vi "eGateHSP_LoadChannelInfo.vi"(7 "path in":path, 8 "Fehler (Eingang, kein Fehler)":errorcluster, 11 "e.gate Configuration":T1 {"StartTime" format="%#.10f"; "dActTimeToSecondFactor" format="%#.10f"; "StartTimeToDayFactor" format="%#_10f"}) -> (0 "Fehler (Ausgang)":errorcluster, 3 "e.gate Configuration 2":T1 {"StartTime" format="%#.10f"; "dActTimeToSecondFactor" format="%#.10f"; "StartTimeToDayFactor" format="%#_10f"})   [LabVIEW 2016]
uses:
  e.gate Configuration.ctl
  e.gate Channel Data.ctl
  e.gate Data Type.ctl
  e.gate Protocol Type.ctl
  e.gate Module  Data.ctl
  e.gateHSP_DLLhandle.ctl
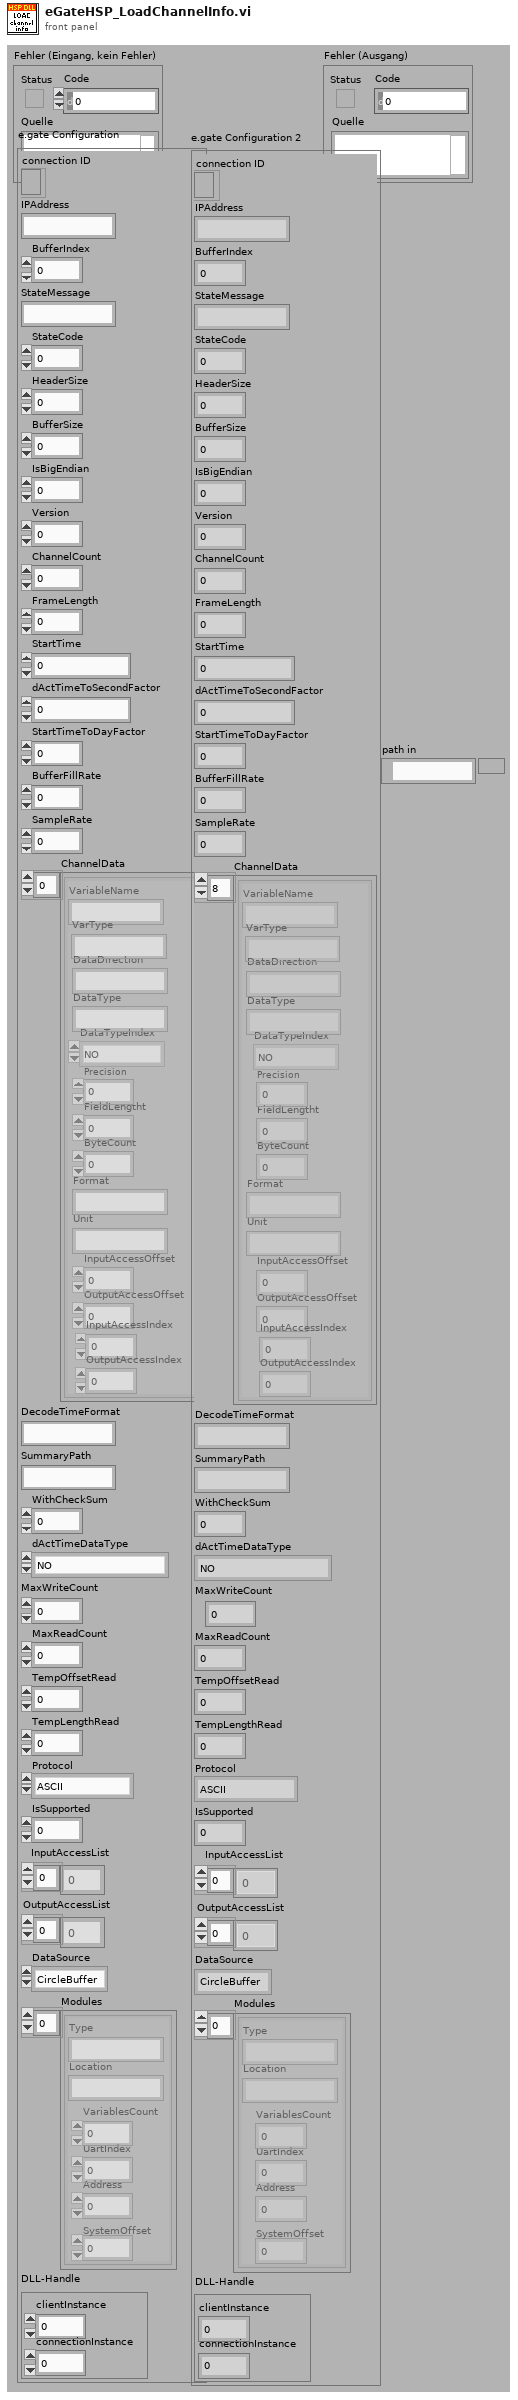
[diagram p1: front panel]
types:
  T1 = typedef "e.gate Configuration.ctl" = cluster{"connection ID":refnum<k5>, "IPAddress":string, "BufferIndex":i32, "StateMessage":string, "StateCode":i8, "HeaderSize":i32, "BufferSize":i32, "IsBigEndian":i32, "Version":i32, "ChannelCount":i32, "FrameLength":i32, "StartTime":dbl, "dActTimeToSecondFactor":dbl, "StartTimeToDayFactor":dbl, "BufferFillRate":dbl, "SampleRate":dbl, "ChannelData":T2[], "DecodeTimeFormat":string, "SummaryPath":string, "WithCheckSum":i32, "dActTimeDataType":T3, "MaxWriteCount":i32, "MaxReadCount":i32, "TempOffsetRead":i32, "TempLengthRead":i32, "Protocol":T4, "IsSupported":i32, "InputAccessList":i32[], "OutputAccessList":i32[], "DataSource":enum16{"CircleBuffer", "test.con Logger", "test.con Archive"}, "Modules":T5[], "DLL-Handle":T6}
  T2 = typedef "e.gate Channel Data.ctl" = cluster{"VariableName":string, "DataDirection":string, "DataType":string, "DataTypeIndex":T3, "Precision":i16, "FieldLengtht":i16, "ByteCount":i32, "Format":string, "Unit":string, "InputAccessOffset":i32, "OutputAccessOffset":i16, "InputAccessIndex":i16, "OutputAccessIndex":i16, "VarType":string}
  T3 = typedef "e.gate Data Type.ctl" = enum16{"NO", "BOOL", "SINT8", "USINT8", "SINT16", "USINT16", "SINT32", "USINT32", "FLOAT", "SET8", "SET16", "SET32", "DOUBLE", "SINT64", "USINT64", "SET64"}
  T4 = typedef "e.gate Protocol Type.ctl" = enum16{"ASCII", "HighspeedPort Online", "HighspeedPort Buffer", "eGateHighspeedPortDLL "}
  T5 = typedef "e.gate Module  Data.ctl" = cluster{"Type":string, "Location":string, "VariablesCount":i16, "UartIndex":i16, "Address":i16, "SystemOffset":i16}
  T6 = typedef "e.gateHSP_DLLhandle.ctl" = cluster{"clientInstance":i32, "connectionInstance":i32}
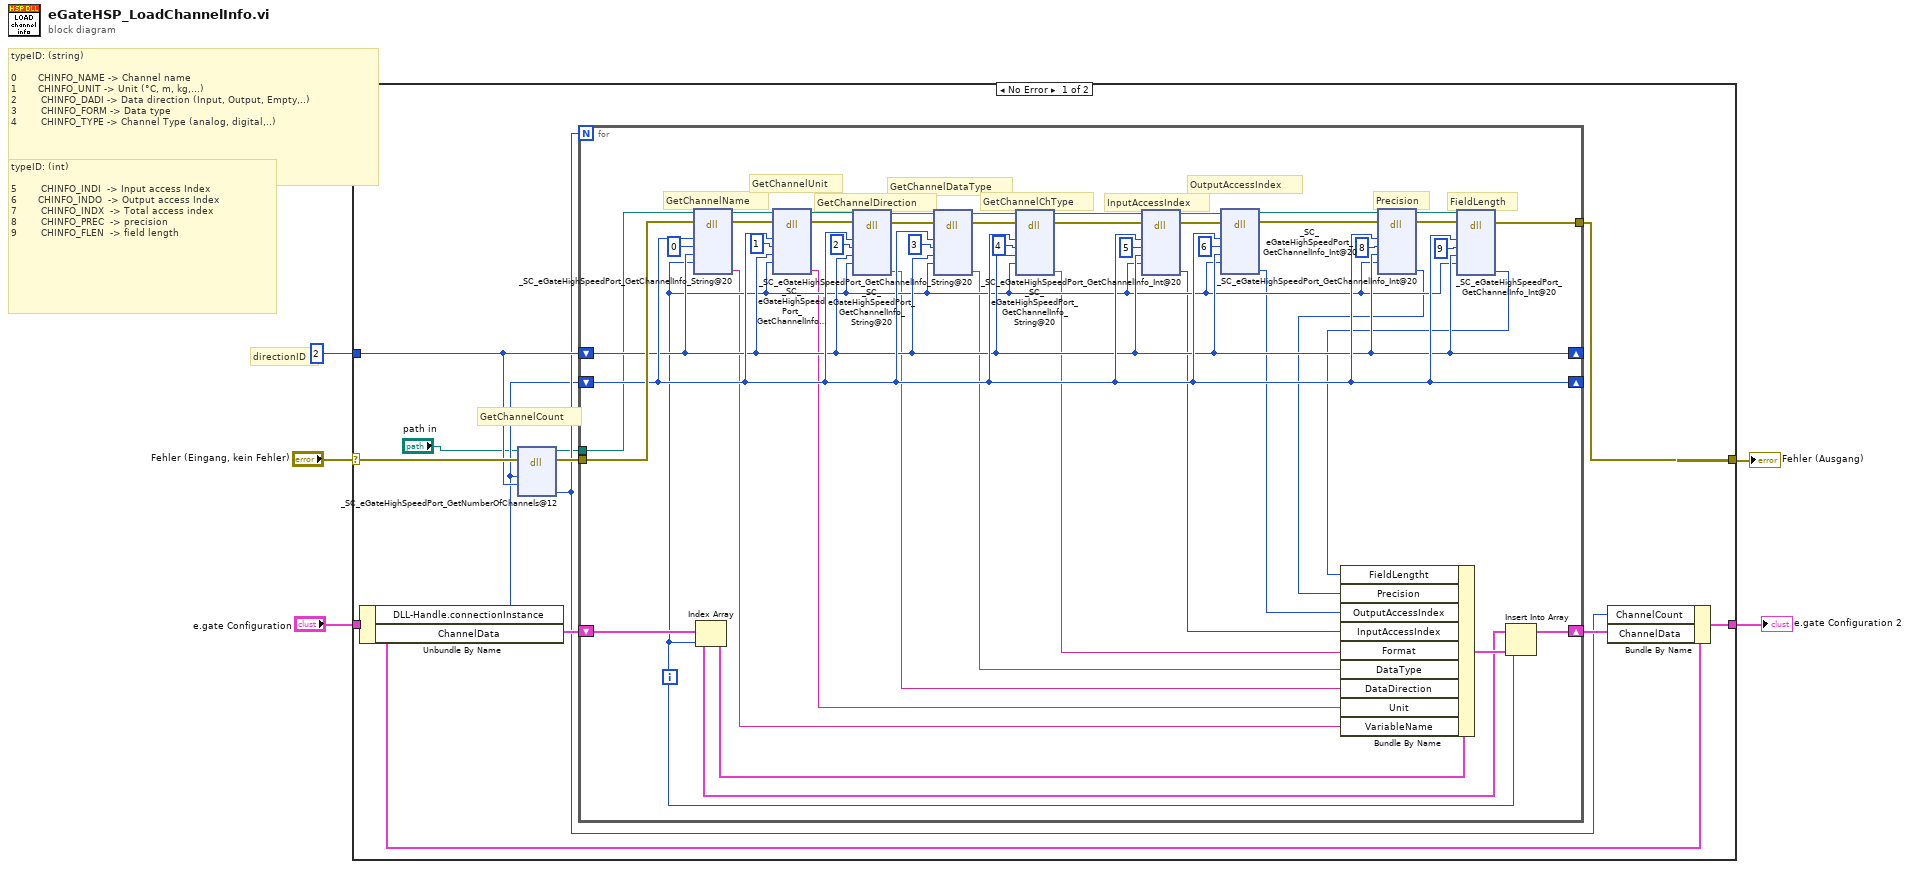
[diagram p0: block diagram]
diagram:
  # "directionID"
  # "typeID: (int)\n\n5\t\t\t\t\t\t\t\tCHINFO_INDI\t\t-> Input access Index\n6\t\t\t\t\t\t\tCHINFO_INDO\t\t-> Output access Index\n7\t\t\t\t\t\t\t\tCHINFO_INDX\t\t-> Total access index\n8\t\t\t\t\t\t\t\tCHINFO_PREC\t\t-> precision\n9\t\t\t\t\t\t\t\tCHINFO_FLEN\t\t-> field length"
  # "typeID: (string)\n\n0\t\t\t\t\t\t\tCHINFO_NAME\t-> Channel name\n1\t\t\t\t\t\t\tCHINFO_UNIT\t-> Unit (°C, m, kg,...)\t\n2\t\t\t\t\t\t\t\tCHINFO_DADI\t-> Data direction (Input, Output, Empty,..)\n3\t\t\t\t\t\t\t\tCHINFO_FORM\t-> Data type\n4\t\t\t\t\t\t\t\tCHINFO_TYPE\t-> Channel Type (analog, digital,..)"
  n1 = case shown="No Error" "Fehler (Eingang, kein Fehler)" {
    selector: "Fehler (Eingang, kein Fehler)" -> [w17 w62]
    tunnel: [w13 w62] -> w4
    tunnel: 2 ("directionID") -> [w14 _]
    tunnel: "e.gate Configuration" -> [w11 _]
    tunnel: [w10 _] -> w2
    frame No Error {
      # "GetChannelCount"
      n2 = Unbundle By Name(w11) -> ("DLL-Handle.connectionInstance"=w8:i32, "ChannelData"=w16:T2[])
      n3 = dll-call lib="eGateHighSpeedPort.dll" fn="_SC_eGateHighSpeedPort_GetNumberOfChannels@12"(path in="path in", error in=w17, "connectionInstance"=w8, "directionID"=w14) -> (path out=w6:path, error out=w15:errorcluster, "ChannelCount"=w9:i32)  [unwired: 5 in]
      n4 = for {
        N: w9 -> [_]
        shift-right: [w59] -> w12
        shift-left: w16 -> [w58]
        tunnel: w15 -> [w51]
        shift-right: [w39] -> _
        shift-left: w8 -> [w39]
        shift-right: [w38] -> _
        shift-left: w14 -> [w38]
        tunnel: [w44] -> w13
        tunnel: w6 -> [w26]
        i -> [w37]
        # "FieldLength"
        # "Precision"
        # "OutputAccessIndex"
        # "InputAccessIndex"
        # "GetChannelChType"
        # "GetChannelDataType"
        # "GetChannelDirection"
        # "GetChannelUnit"
        # "GetChannelName"
        n5 = dll-call lib="eGateHighSpeedPort.dll" fn="_SC_eGateHighSpeedPort_GetChannelInfo_String@20"(path in=w26, error in=w51, "connectionInstance"=w39, "typeID"=0, "directionID"=w38, "channelIndex"=w37) -> (path out=w25:path, error out=w56:errorcluster, "ChannelInfo"=w35:string)  [unwired: 7 in]
        n6 = Index Array(array=w58, index=w37) -> (element=w61:T2)
        n7 = dll-call lib="eGateHighSpeedPort.dll" fn="_SC_eGateHighSpeedPort_GetChannelInfo_String@20"(path in=w25, error in=w56, "connectionInstance"=w39, "typeID"=1, "directionID"=w38, "channelIndex"=w37) -> (path out=w24:path, error out=w50:errorcluster, "ChannelInfo"=w34:string)  [unwired: 7 in]
        n8 = dll-call lib="eGateHighSpeedPort.dll" fn="_SC_eGateHighSpeedPort_GetChannelInfo_String@20"(path in=w24, error in=w50, "connectionInstance"=w39, "typeID"=2, "directionID"=w38, "channelIndex"=w37) -> (path out=w23:path, error out=w49:errorcluster, "ChannelInfo"=w33:string)  [unwired: 7 in]
        n9 = dll-call lib="eGateHighSpeedPort.dll" fn="_SC_eGateHighSpeedPort_GetChannelInfo_String@20"(path in=w23, error in=w49, "connectionInstance"=w39, "typeID"=3, "directionID"=w38, "channelIndex"=w37) -> (path out=w22:path, error out=w48:errorcluster, "ChannelInfo"=w32:string)  [unwired: 7 in]
        n10 = dll-call lib="eGateHighSpeedPort.dll" fn="_SC_eGateHighSpeedPort_GetChannelInfo_String@20"(path in=w22, error in=w48, "connectionInstance"=w39, "typeID"=4, "directionID"=w38, "channelIndex"=w37) -> (path out=w21:path, error out=w47:errorcluster, "ChannelInfo"=w31:string)  [unwired: 7 in]
        n11 = dll-call lib="eGateHighSpeedPort.dll" fn="_SC_eGateHighSpeedPort_GetChannelInfo_Int@20"(path in=w21, error in=w47, "connectionInstance"=w39, "typeID"=5, "directionID"=w38, "channelIndex"=w37) -> (path out=w20:path, error out=w46:errorcluster, "ChannelInfo"=w30:i32)  [unwired: 7 in]
        n12 = dll-call lib="eGateHighSpeedPort.dll" fn="_SC_eGateHighSpeedPort_GetChannelInfo_Int@20"(path in=w20, error in=w46, "connectionInstance"=w39, "typeID"=6, "directionID"=w38, "channelIndex"=w37) -> (path out=w19:path, error out=w36:errorcluster, "ChannelInfo"=w29:i32)  [unwired: 7 in]
        n13 = dll-call lib="eGateHighSpeedPort.dll" fn="_SC_eGateHighSpeedPort_GetChannelInfo_Int@20"(path in=w19, error in=w36, "connectionInstance"=w39, "typeID"=8, "directionID"=w38, "channelIndex"=w37) -> (path out=w18:path, error out=w45:errorcluster, "ChannelInfo"=w28:i32)  [unwired: 7 in]
        n14 = dll-call lib="eGateHighSpeedPort.dll" fn="_SC_eGateHighSpeedPort_GetChannelInfo_Int@20"(path in=w18, error in=w45, "connectionInstance"=w39, "typeID"=9, "directionID"=w38, "channelIndex"=w37) -> (error out=w44:errorcluster, "ChannelInfo"=w27:i32)  [unwired: 7 in, 1 out]
        n15 = Bundle By Name(cluster=w61, "FieldLengtht"=w27, "Precision"=w28, "OutputAccessIndex"=w29, "InputAccessIndex"=w30, "Format"=w31, "DataType"=w32, "DataDirection"=w33, "Unit"=w34, "VariableName"=w35) -> (w60:T2)
        n16 = Insert Into Array(array=w58, index=w37, new element=w60) -> (w59:T2[])
      }
      n17 = Bundle By Name(cluster=w11, "ChannelCount"=w9, "ChannelData"=w12) -> (w10:T1)
    }
    frame Error {
    }
  }
  "Fehler (Ausgang)" <- w4
  "e.gate Configuration 2" <- w2
